vi "Instantiate.vi"(1 "vi ref":refnum<vi>) -> (0 "vi ref":refnum<vi>)   [LabVIEW 2020, in "Flex.lvlib"]
doc: "Creates and initializes the data structure that supports the channel at run time."
uses:
  Flex.lvlib
  ChannelOp.ctl
  ))Channel.vi
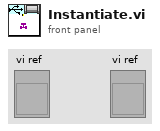
[diagram p1: front panel]
types:
  T1 = typedef "Flex.lvlib/ChannelOp.ctl" = enum16{"Get Refs", "Init", "Close", "Probe", "New Queue", "Remove Queue"}
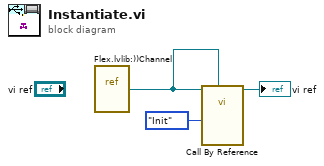
[diagram p0: block diagram]
diagram:
  n1 = vi-ref "Flex.lvlib:))Channel.vi"() -> (w2:refnum<vi>)
  n2 = call-by-ref "?"(reference=w2, "This VI"=w2, "channelOp"=ChannelOp."Init") -> (reference out=→"vi ref":refnum<vi>)  [unwired: 7 in, 5 out]
